vi "Calc_Regression_Metrics.vi"(6 "Dataset":T2={"Inputs Ref."=variant(refnum<data-value> refnum), "Outputs Ref."=refnum, "Dataset_Size"=0, "Dims_In"={"C"=0, "H"=0, "W"=0}, "Dims_Out"=0, "Labels"=[], "File Paths"=[]}, 11 "Predictions":sgl[][](array[numeric])) -> (3 "Metrics":T1 {"R" format="%#_7g"})   [LabVIEW 2020]
uses:
  <vilib>/Ngene/Deep Learning Toolkit/Toolkit/NN_Data/API/DataSet/DataSet_Types/NN_DataSet(In3D_Out1D).ctl
  <vilib>/Ngene/Deep Learning Toolkit/Toolkit/NN_Data/Controls/DataRef_Types/2D/NN_Data_ref(2D_SGL).ctl
  <vilib>/Ngene/Deep Learning Toolkit/Toolkit/NN_Data/API/NN_Dims(C,H,W).ctl
  Controls/Regression_Report.ctl
  <vilib>/Analysis/baseanly.llb/Mean (DBL).vi
  <vilib>/Ngene/Deep Learning Toolkit/Toolkit/NN_Data/subVIs/Get_Data_Vals/2D/NN_Data_Get_ValByRef(2D_SGL).vi
  <vilib>/Analysis/NI_AALBase.lvlib
  <vilib>/Ngene/Deep Learning Toolkit/Toolkit/Deep_Learning_Toolkit_by_Ngene.lvlib
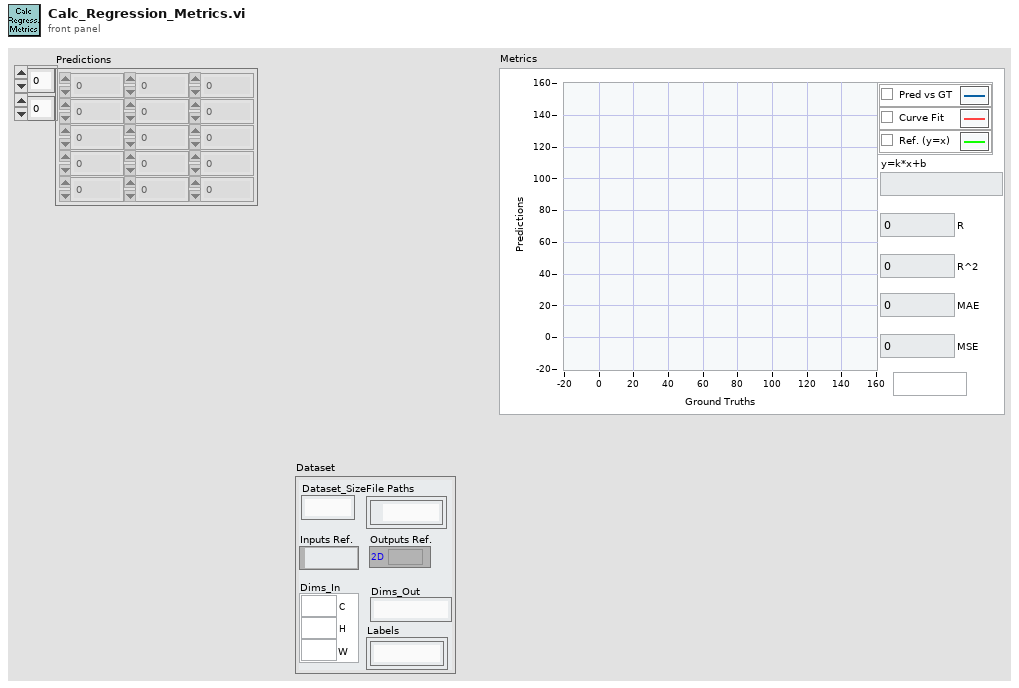
[diagram p1: front panel]
types:
  T1 = typedef "Regression_Report.ctl" = cluster{"Graphs":cluster{"Best Linear Fit":dbl[], "Array 3":sgl[]}[], "y=k*x+b":string, "R":sgl, "R^2":sgl, "MAE":sgl, "MSE":sgl}
  T2 = typedef "Deep_Learning_Toolkit_by_Ngene.lvlib/NN_DataSet(In3D_Out1D).ctl" = cluster{"Inputs Ref.":variant, "Outputs Ref.":T3, "Dataset_Size":i32, "Dims_In":T4, "Dims_Out":i32, "Labels":string[], "File Paths":path[]}
  T3 = typedef "Deep_Learning_Toolkit_by_Ngene.lvlib/NN_Data_ref(2D_SGL).ctl" = refnum<data-value>
  T4 = typedef "Deep_Learning_Toolkit_by_Ngene.lvlib/NN_Dims(C,H,W).ctl" = cluster{"C":i32, "H":i32, "W":i32}
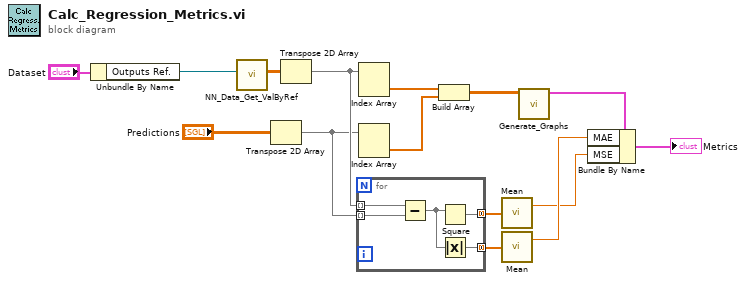
[diagram p0: block diagram]
diagram:
  n1 = Unbundle By Name("Dataset") -> ("Outputs Ref."=w9:T3)
  n2 = call-poly <vilib>:"NN_Data_Get_ValByRef.vi"("DVR(2D_SGL)"=w9) -> ("Value(2D_SGL)"=w8:sgl[][])  [unwired: 7 in, 1 out]
  n3 = Transpose 2D Array(2D array="Predictions") -> (transposed array=w10:sgl[][])
  n4 = Transpose 2D Array(2D array=w8) -> (transposed array=w11:sgl[][])
  n5 = for {
    tunnel: w11 -> [w17] mode=indexing
    tunnel: w10 -> [w16] mode=indexing
    tunnel: [w20] -> w13 mode=concatenating
    tunnel: [w18] -> w12 mode=concatenating
    n6 = Subtract(x=w17, y=w16) -> (x-y=w19:sgl[])
    n7 = Square(x=w19) -> (x^2=w20:sgl[])
    n8 = Absolute Value(x=w19) -> (abs(x)=w18:sgl[])
  }
  n9 = Index Array(array=w11) -> (element=w7:sgl[])  [unwired: 2 in]
  n10 = Index Array(array=w10) -> (element=w6:sgl[])  [unwired: 2 in]
  n11 = Build Array(w7, w6) -> (w5:sgl[][])
  n12 = call-poly <vilib>:"Mean.vi"("X"=w13) -> ("mean"=w1:dbl)  [unwired: 1 out]
  n13 = call-poly <vilib>:"Mean.vi"("X"=w12) -> ("mean"=w2:dbl)  [unwired: 1 out]
  n14 = call "Generate_Graphs.vi"("Data (GT, Pred)"=w5) -> ("Report"=w4:T1)  [unwired: 10 in]
  n15 = Bundle By Name(cluster=w4, "MAE"=w2, "MSE"=w1) -> (→"Metrics":T1)
